vi "[FPGA] DeltaSig Main V6_bis.vi"() -> ()   [LabVIEW 2015]
doc: "This VI provides a template for customizing a waveform acquisition using delta-sigma based NI C Series analog input smodules."
uses:
  <vilib>/LabVIEW Targets/FPGA/cRIO/shared/nicrio_ModuleControls/nicrio_cRIO-9234_ConfigModeRing.ctl
  <vilib>/rvi/Emulation/niFpgaGetClockAttributes.vi
  <vilib>/rvi/Emulation/niFpgaSctlEmulationGetInTimedLoop.vi
  <vilib>/rvi/Emulation/niFpgaEmulationReportErrorSimple.vi
  <vilib>/LabVIEW Targets/FPGA/cRIO/shared/nicrio_DsaDataRateApi/_nicrio_9234GetDataRate131.vi
  <vilib>/rvi/Emulation/niFpgaProcessEmulError.vi
  <vilib>/rvi/eio/common/nirviEmuTemplatePropertySet_errors.vi
  <vilib>/rvi/eio/common/nirviEmuTemplateMethod_errors.vi
  <vilib>/rvi/interface/RandomDataEmulation/niFpgaRandomDataHandleErrors.vi
  <vilib>/rvi/Emulation/niFpgaCriticalErrorInLSC.vi
  <vilib>/eio/EIOPropertyNode/EIOPropertyNode.xnode
  <vilib>/LabVIEW Targets/FPGA/cRIO/shared/nicrio_ModuleControls/nicrio_cRIO-9234_DataRatesRing2.ctl
  <vilib>/eio/EIONode/EIONode.xnode
  <vilib>/rvi/DataTransferAndStorage/Container/XNode/niFpgaContainer.xnode
  <vilib>/rvi/interface/RandomDataEmulation/nirviRandomDataFpgaReadWriteTemplate.vi
  <vilib>/rvi/eio/common/nirviEmuTemplatePropertyGet_errors.vi
  <vilib>/rvi/eio/common/nirviEmuTemplatePropertyGet_noerrors.vi
  <vilib>/rvi/eio/common/nirviEmuTemplatePropertySet_noerrors.vi
panel:
  in  "Array Input Config":T1[](array[typedef])=[0, 0, 0, 0, 0, 0] items=["AC Coupled", "DC Coupled", "IEPE AC Coupled"]
  out "oclk freq":u32
  out "oclk div":u32
  out "oclk mult":u32
  in  "data rate (S/s)":u32
  in  "Chan Scale Array":sgl[](array[numeric])=[0.0, 0.0, 0.0, 0.0, 0.0, 0.0, 0.0, 0.0, 0.0, 0.0, 0.0, 0.0, 0.0, 0.0, 0.0, 0.0, 0.0, 0.0, 0.0, 0.0, 0.0, 0.0, 0.0, 0.0, 0.0, 0.0, 0.0, 0.0, 0.0, 0.0, 0.0, 0.0, 0.0, 0.0, 0.0, 0.0, 0.0, 0.0, 0.0, 0.0]
  out "Chan Count":bool
  out "Acq Loop Ticks":u32
  out "FPGA Error":errorcluster
  out "Module Underflow":bool
  out "Finished":bool
  in  "Number of Channels":i32=24
  in  "Samps per Chan [Finite]":i32=5120
  out "First Read":bool
  in  "Acquisition Type":enum16{"Finite Samples", "Continuous Samples"}(ring)
  out "DMA FIFO Full":bool
  in  "stop":bool
  # "Array size fixed at 40\nelements but may be \nexpanded if needed"
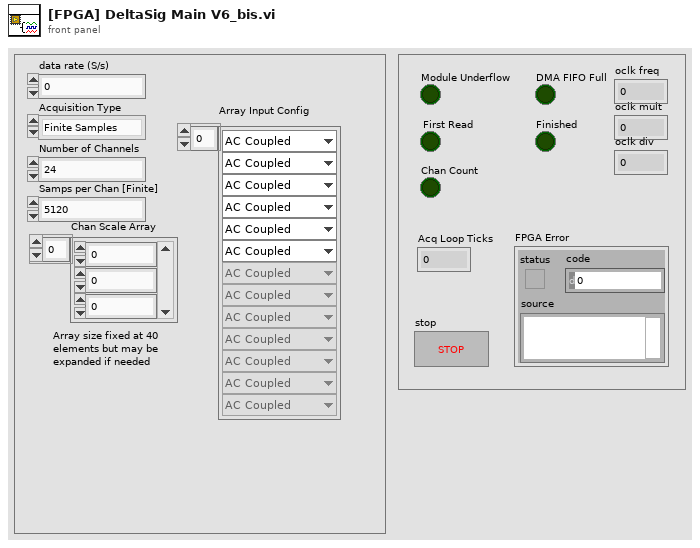
[diagram p1: front panel]
types:
  T1 = typedef "nicrio_cRIO-9234_ConfigModeRing.ctl" = u8
  T2 = typedef "nicrio_cRIO-9234_DataRatesRing2.ctl" = u8
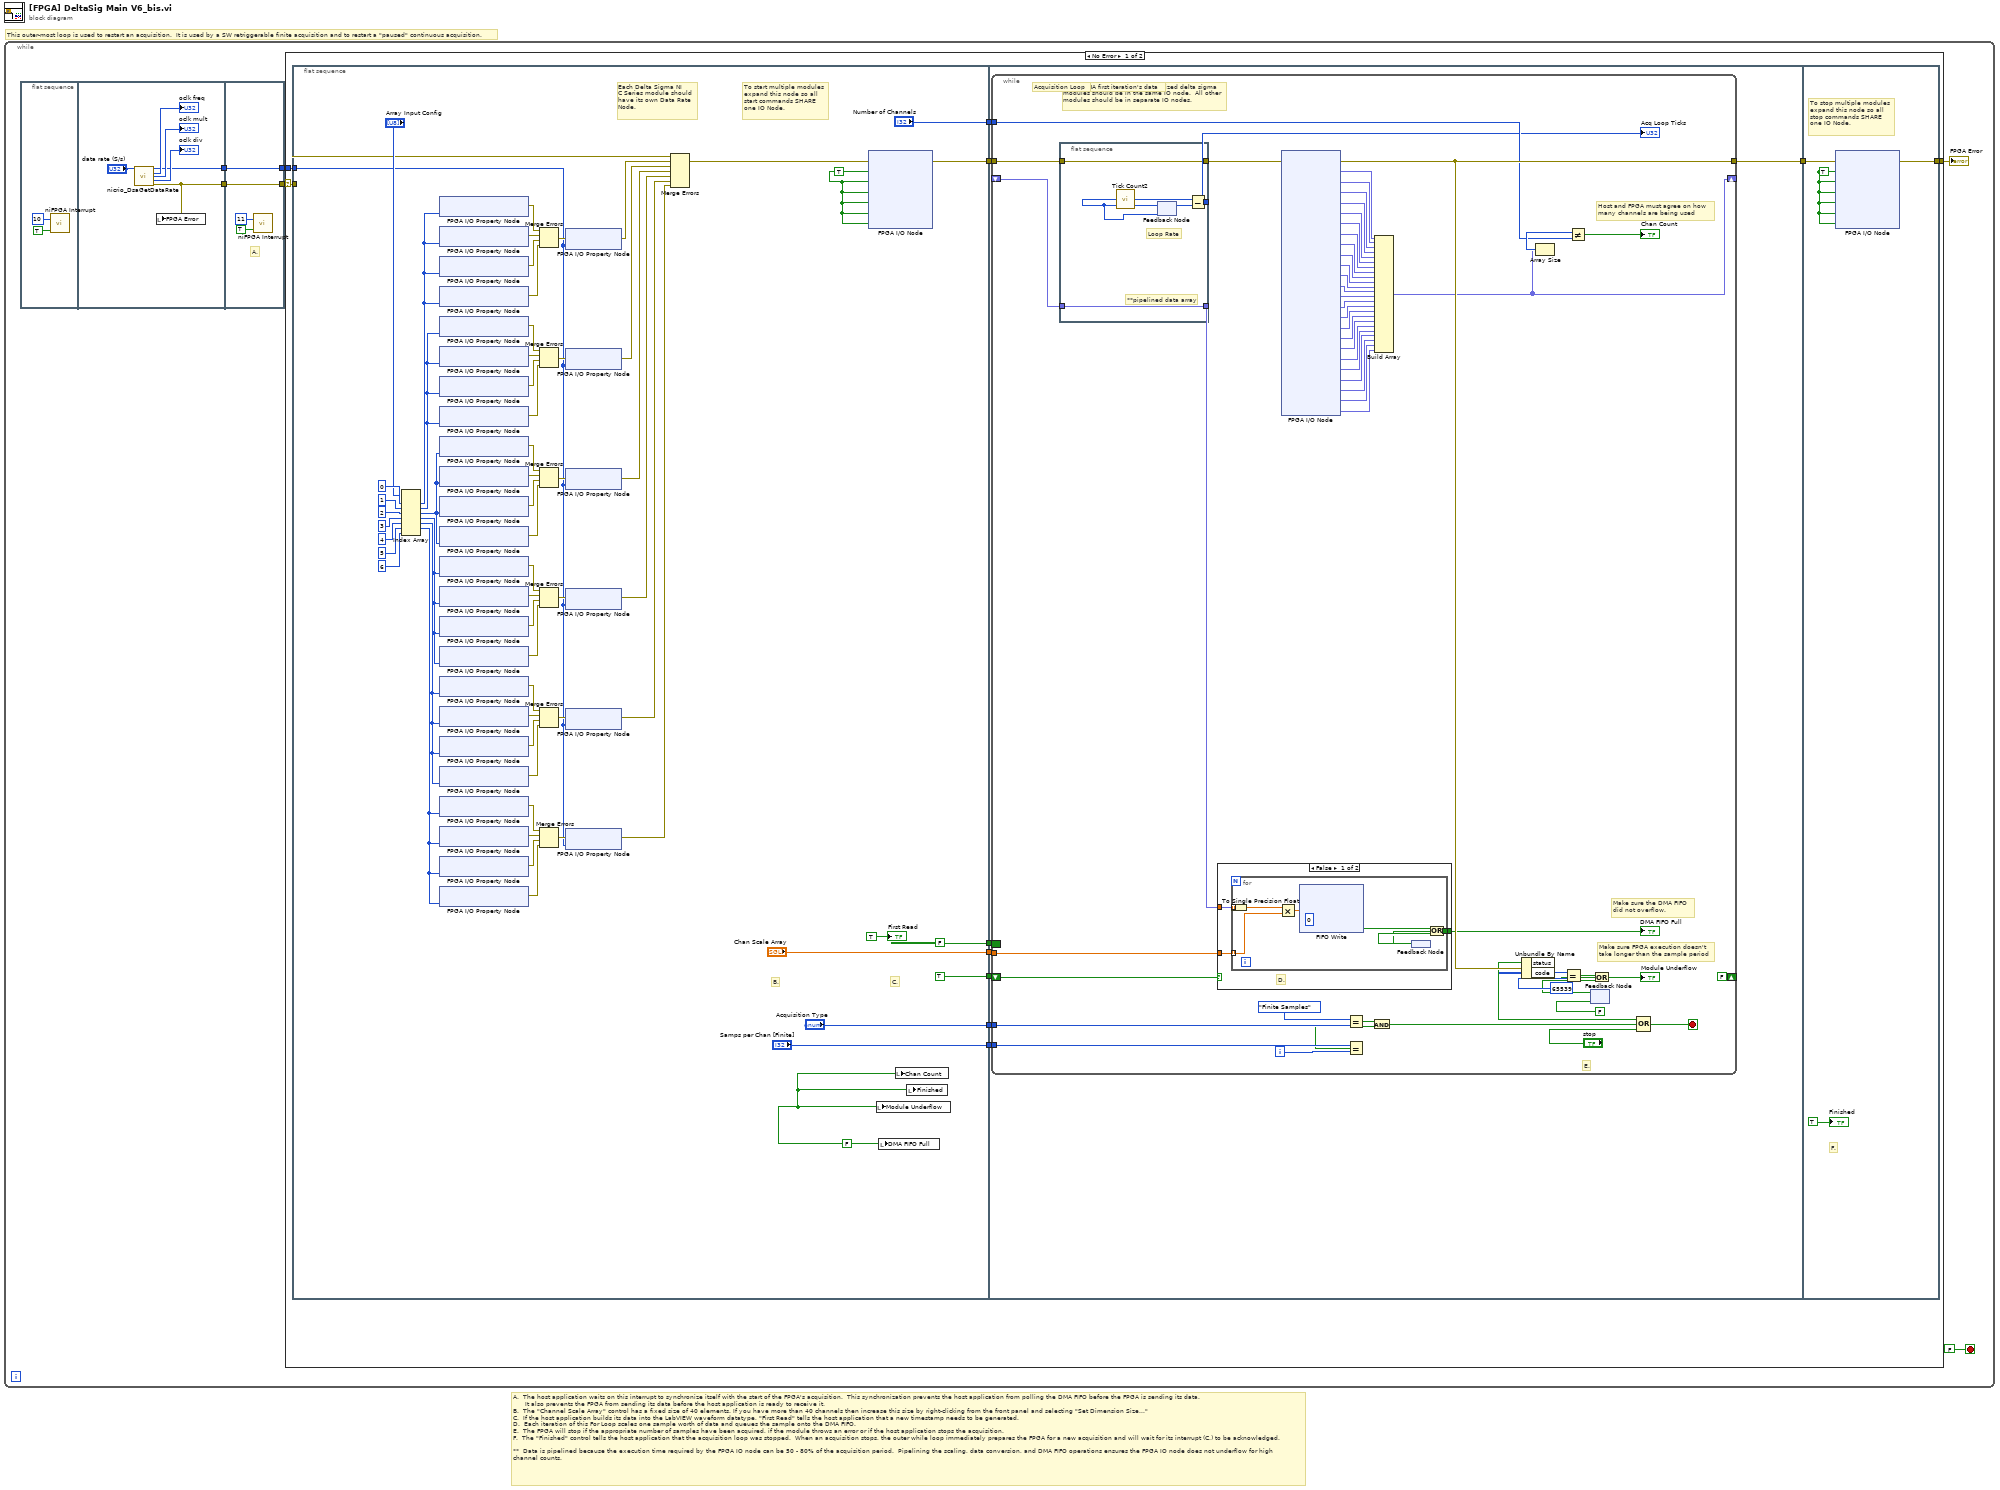
[diagram p0: block diagram]
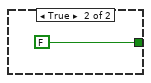
[diagram p2: hidden frame]
diagram:
  # "A.  The host application waits on this interrupt to synchronize itself with the start of the FPGA's acquisition.  This synchronization prevents the host application from polling the DMA FIFO before the FPGA is sending its data.\n      It also prevents the FPGA from sending its data before the host application is ready to receive it.\nB.  The \"Channel Scale Array\" control has a fixed size of 40 elements. If you have more than 40 channels then increase this size by right-clicking from the front panel and selecting \"Set Dimension Size...\"\nC.  If the host application builds its data into the LabVIEW waveform datatype, \"First Read\" tells the host application that a new timestamp needs to be generated.\nD.  Each iteration of this For Loop scales one sample worth of data and queues the sample onto the DMA FIFO.  \nE.  The FPGA will stop if the appropriate number of samples have been acquired, if the module throws an error or if the host application stops the acquisition.  \nF.  The \"Finished\" control tells the host application that the acquisition loop was stopped.  When an acquisition stops, the outer while loop immediately prepares the FPGA for a new acquisition and will wait for its interrupt (C.) to be acknowledged.\n\n**  Data is pipelined because the execution time required by the FPGA IO node can be 50 - 80% of the acquisition period.  Pipelining the scaling, data conversion, and DMA FIFO operations ensures the FPGA IO node does not underflow for high\nchannel counts."
  # "This outer-most loop is used to restart an acquisition.  It is used by a SW retriggerable finite acquisition and to restart a \"paused\" continuous acquisition."
  n1 = while {
    stop <- FALSE stop-if-true
    n2 = flat-sequence {
      tunnel: [w10] -> w2
      tunnel: [w11] -> w1
      tunnel: [w18] -> w3
      tunnel: [w15] -> w4
      tunnel: w2 -> [w15]
      tunnel: w1 -> [w18]
      frame #0 {
        n3 = call <vilib>:"niFPGA Interrupt.vi"("Wait Until Cleared (F)"=TRUE ("Wait Until Cleared"), "IRQ Number (0)"=u8 10 ("IRQ Number")) -> ()  [unwired: 1 in]
      }
      frame #1 {
        n4 = call-poly <vilib>:"nicrio_DsaGetDataRate.vi"("data rate (S/s)"="data rate (S/s)") -> ("data rate"=w11:T2, "oclk freq"=→"oclk freq":u32, "oclk mult"=→"oclk mult":u32, "oclk div"=→"oclk div":u32, "error out"=w10:errorcluster)  [unwired: 10 in]
        n5 = local write "FPGA Error"(w10) -> ()
      }
      frame #2 {
        # "A."
        n6 = call <vilib>:"niFPGA Interrupt.vi"("Wait Until Cleared (F)"=TRUE ("Wait Until Cleared"), "IRQ Number (0)"=u8 11 ("IRQ Number")) -> ()  [unwired: 1 in]
      }
    }
    n7 = case shown="No Error" w4 {
      selector: w4 -> [w19 w176]
      tunnel: [w21 w176] -> w5
      tunnel: w3 -> [w20 _]
      frame No Error {
        n8 = flat-sequence {
          tunnel: [w92] -> w29
          tunnel: ["Chan Scale Array"] -> w28
          tunnel: ["Acquisition Type"] -> w27
          tunnel: ["Samps per Chan [Finite]"] -> w26
          tunnel: ["Number of Channels"] -> w25
          tunnel: [TRUE ("t")] -> w24
          tunnel: [FALSE] -> w23
          tunnel: w20 -> [w38]
          tunnel: w19 -> [w68]
          tunnel: w29 -> [w99]
          tunnel: w28 -> [w98]
          tunnel: w27 -> [w96]
          tunnel: w26 -> [w95]
          tunnel: w25 -> [w100]
          tunnel: w24 -> [w97]
          tunnel: [w94] -> w22
          tunnel: w23 -> [w93]
          tunnel: w22 -> [w174]
          tunnel: [w173] -> w21
          frame #0 {
            w90 = FALSE ("Module Underflow")
            w30 = TRUE ("Mod1/Start")
            # "To start multiple modules\nexpand this node so all\nstart commands SHARE\none IO Node."
            # "C."
            # "B."
            # "Each Delta Sigma NI \nC Series module should \nhave its own Data Rate \nNode."
            n9 = Index Array(array="Array Input Config", index #1=0 ("index"), index #2=1 ("index"), index #3=2 ("index"), index #4=3 ("index"), index #5=4 ("index"), index #6=5 ("index"), index #7=6 ("index")) -> (element #1=w36:T1, element #2=w35:T1, element #3=w34:T1, element #4=w33:T1, element #5=w32:T1, element #6=w31:T1)  [unwired: 1 out]
            n10 = xnode "FPGA I/O Property Node"("Input Configuration"=w36) -> ("error out"=w79:errorcluster)  [unwired: 2 in, 1 out]
            n11 = xnode "FPGA I/O Property Node"("Input Configuration"=w36) -> ("error out"=w78:errorcluster)  [unwired: 2 in, 1 out]
            n12 = xnode "FPGA I/O Property Node"("Input Configuration"=w36) -> ("error out"=w77:errorcluster)  [unwired: 2 in, 1 out]
            n13 = xnode "FPGA I/O Property Node"("Input Configuration"=w36) -> ("error out"=w76:errorcluster)  [unwired: 2 in, 1 out]
            n14 = xnode "FPGA I/O Property Node"("Input Configuration"=w35) -> ("error out"=w73:errorcluster)  [unwired: 2 in, 1 out]
            n15 = xnode "FPGA I/O Property Node"("Input Configuration"=w35) -> ("error out"=w72:errorcluster)  [unwired: 2 in, 1 out]
            n16 = xnode "FPGA I/O Property Node"("Input Configuration"=w35) -> ("error out"=w71:errorcluster)  [unwired: 2 in, 1 out]
            n17 = xnode "FPGA I/O Property Node"("Input Configuration"=w35) -> ("error out"=w70:errorcluster)  [unwired: 2 in, 1 out]
            n18 = xnode "FPGA I/O Property Node"("Input Configuration"=w34) -> ("error out"=w61:errorcluster)  [unwired: 2 in, 1 out]
            n19 = xnode "FPGA I/O Property Node"("Input Configuration"=w34) -> ("error out"=w60:errorcluster)  [unwired: 2 in, 1 out]
            n20 = xnode "FPGA I/O Property Node"("Input Configuration"=w34) -> ("error out"=w59:errorcluster)  [unwired: 2 in, 1 out]
            n21 = xnode "FPGA I/O Property Node"("Input Configuration"=w34) -> ("error out"=w58:errorcluster)  [unwired: 2 in, 1 out]
            n22 = xnode "FPGA I/O Property Node"("Input Configuration"=w33) -> ("error out"=w57:errorcluster)  [unwired: 2 in, 1 out]
            n23 = xnode "FPGA I/O Property Node"("Input Configuration"=w33) -> ("error out"=w56:errorcluster)  [unwired: 2 in, 1 out]
            n24 = xnode "FPGA I/O Property Node"("Input Configuration"=w33) -> ("error out"=w55:errorcluster)  [unwired: 2 in, 1 out]
            n25 = xnode "FPGA I/O Property Node"("Input Configuration"=w33) -> ("error out"=w54:errorcluster)  [unwired: 2 in, 1 out]
            n26 = xnode "FPGA I/O Property Node"("Input Configuration"=w32) -> ("error out"=w53:errorcluster)  [unwired: 2 in, 1 out]
            n27 = xnode "FPGA I/O Property Node"("Input Configuration"=w32) -> ("error out"=w52:errorcluster)  [unwired: 2 in, 1 out]
            n28 = xnode "FPGA I/O Property Node"("Input Configuration"=w32) -> ("error out"=w51:errorcluster)  [unwired: 2 in, 1 out]
            n29 = xnode "FPGA I/O Property Node"("Input Configuration"=w32) -> ("error out"=w50:errorcluster)  [unwired: 2 in, 1 out]
            n30 = xnode "FPGA I/O Property Node"("Input Configuration"=w31) -> ("error out"=w39:errorcluster)  [unwired: 2 in, 1 out]
            n31 = xnode "FPGA I/O Property Node"("Input Configuration"=w31) -> ("error out"=w43:errorcluster)  [unwired: 2 in, 1 out]
            n32 = xnode "FPGA I/O Property Node"("Input Configuration"=w31) -> ("error out"=w42:errorcluster)  [unwired: 2 in, 1 out]
            n33 = xnode "FPGA I/O Property Node"("Input Configuration"=w31) -> ("error out"=w41:errorcluster)  [unwired: 2 in, 1 out]
            n34 = Merge Errors(w79, w78, w77, w76) -> (w75:errorcluster)
            n35 = Merge Errors(w73, w72, w71, w70) -> (w69:errorcluster)
            n36 = Merge Errors(w61, w60, w59, w58) -> (w49:errorcluster)
            n37 = Merge Errors(w57, w56, w55, w54) -> (w48:errorcluster)
            n38 = Merge Errors(w53, w52, w51, w50) -> (w47:errorcluster)
            n39 = Merge Errors(w39, w43, w42, w41) -> (w40:errorcluster)
            n40 = xnode "FPGA I/O Property Node"("error in"=w75, "Data Rate"=w38) -> ("error out"=w66:errorcluster)  [unwired: 1 in, 1 out]
            n41 = xnode "FPGA I/O Property Node"("error in"=w69, "Data Rate"=w38) -> ("error out"=w65:errorcluster)  [unwired: 1 in, 1 out]
            n42 = xnode "FPGA I/O Property Node"("error in"=w49, "Data Rate"=w38) -> ("error out"=w46:errorcluster)  [unwired: 1 in, 1 out]
            n43 = xnode "FPGA I/O Property Node"("error in"=w48, "Data Rate"=w38) -> ("error out"=w45:errorcluster)  [unwired: 1 in, 1 out]
            n44 = xnode "FPGA I/O Property Node"("error in"=w47, "Data Rate"=w38) -> ("error out"=w44:errorcluster)  [unwired: 1 in, 1 out]
            n45 = xnode "FPGA I/O Property Node"("error in"=w40, "Data Rate"=w38) -> ("error out"=w37:errorcluster)  [unwired: 1 in, 1 out]
            n46 = Merge Errors(w68, w66, w65, w46, w45, w44, w37) -> (w67:errorcluster)
            n47 = xnode "FPGA I/O Node"("error in"=w67, "Mod1/Start"=w30, "Mod2/Start"=w30, "Mod3/Start"=w30, "Mod4/Start"=w30, "Mod5/Start"=w30, "Mod6/Start"=w30) -> ("error out"=w92:errorcluster)  [unwired: 6 in, 6 out]
            n48 = local write "Module Underflow"(w90) -> ()
            n49 = local write "DMA FIFO Full"(w90) -> ()
            n50 = local write "Chan Count"(w90) -> ()
            n51 = local write "Finished"(w90) -> ()
            "First Read" <- TRUE ("First Read")
          }
          frame #1 {
            n52 = while {
              tunnel: w99 -> [w144]
              tunnel: [w149] -> w94
              tunnel: w96 -> [w151]
              tunnel: w95 -> [w150]
              shift-right: [w124] -> _
              shift-left: _ -> [w137]
              tunnel: w100 -> [w146]
              tunnel: w98 -> [w138]
              shift-right: [FALSE ("t")] -> _
              shift-left: w97 -> [w136]
              border: w93 -> [_]
              i -> [w134]
              stop <- w121 stop-if-true
              # "Add channels here.  All synchronized delta sigma\nmodules should be in the same IO node.  All other\nmodules should be in separate IO nodes."
              # "Do not DMA first iteration's data"
              # "Acquisition Loop"
              # "E."
              # "Host and FPGA must agree on how \nmany channels are being used"
              # "Make sure the DMA FIFO\ndid not overflow."
              # "Make sure FPGA execution doesn't\ntake longer than the sample period"
              n53 = flat-sequence {
                tunnel: [w171] -> w143
                tunnel: w144 -> [w171]
                tunnel: [w168] -> w142
                tunnel: w137 -> [w167]
                tunnel: [w167] -> w123
                frame #0 {
                  # "**pipelined data array"
                  # "Loop Rate"
                  n54 = call "Tick Count2"() -> ("Tick Count(Ticks)"=w170:u32)
                  n55 = feedback-in #1(w170) -> ()
                  n56 = feedback #1(w170) -> (w169:u32)
                  n57 = Subtract(x=w170, y=w169) -> (x-y=w168:u32)
                }
              }
              n58 = To Single Precision Float(number=w123) -> (single precision float=w122:sgl[])
              n59 = case shown="False" w136 {
                tunnel: [w158 FALSE] -> w148
                tunnel: w138 -> [w157 _]
                tunnel: w122 -> [w156 _]
                frame False {
                  # "D."
                  n60 = for {
                    tunnel: [w163] -> w158
                    tunnel: w156 -> [w161] mode=indexing
                    tunnel: w157 -> [w160] mode=indexing
                    n61 = Multiply(x=w161, y=w160) -> (x*y=w159:sgl)
                    n62 = xnode ("FIFO Write")("Element"=w159, "Timeout"=0) -> ("Timed Out?"=w165:bool)  [unwired: 1 in, 1 out]
                    n63 = feedback #2() -> (w164:bool)
                    n64 = Or(x=w165, y=w164) -> (x .or. y?=w163:bool)
                    n65 = feedback-in #2(w163) -> ()
                  }
                }
                frame True {
                }
              }
              "DMA FIFO Full" <- w148
              n66 = xnode "FPGA I/O Node"("error in"=w143) -> ("error out"=w149:errorcluster, "Mod1/AI0"=w141:fxp<+/-,24,4>, "Mod1/AI1"=w133:fxp<+/-,24,4>, "Mod1/AI2"=w140:fxp<+/-,24,4>, "Mod1/AI3"=w139:fxp<+/-,24,4>, "Mod2/AI0"=w120:fxp<+/-,24,4>, "Mod2/AI1"=w119:fxp<+/-,24,4>, "Mod2/AI2"=w118:fxp<+/-,24,4>, "Mod2/AI3"=w117:fxp<+/-,24,4>, "Mod3/AI0"=w116:fxp<+/-,24,4>, "Mod3/AI1"=w115:fxp<+/-,24,4>, "Mod3/AI2"=w114:fxp<+/-,24,4>, "Mod3/AI3"=w113:fxp<+/-,24,4>, "Mod4/AI0"=w112:fxp<+/-,24,4>, "Mod4/AI1"=w111:fxp<+/-,24,4>, "Mod4/AI2"=w110:fxp<+/-,24,4>, "Mod4/AI3"=w109:fxp<+/-,24,4>, "Mod5/AI0"=w108:fxp<+/-,24,4>, "Mod5/AI1"=w107:fxp<+/-,24,4>, "Mod5/AI2"=w106:fxp<+/-,24,4>, "Mod5/AI3"=w105:fxp<+/-,24,4>, "Mod6/AI0"=w104:fxp<+/-,24,4>, "Mod6/AI1"=w103:fxp<+/-,24,4>, "Mod6/AI2"=w102:fxp<+/-,24,4>, "Mod6/AI3"=w101:fxp<+/-,24,4>)  [unwired: 24 in, 24 out]
              n67 = Equal?(x=enum16{"Finite Samples", "Continuous Samples"}."Finite Samples" ("y"), y=w151) -> (x = y?=w127:bool)
              n68 = Equal?(x=w150, y=w134) -> (x = y?=w126:bool)
              n69 = And(x=w127, y=w126) -> (x .and. y?=w125:bool)
              n70 = Build Array(w141, w133, w140, w139, w120, w119, w118, w117, w116, w115, w114, w113, w112, w111, w110, w109, w108, w107, w106, w105, w104, w103, w102, w101) -> (w124:fxp<+/-,24,4>[])
              n71 = Unbundle By Name(w149) -> ("status"=w132:bool, "code"=w152:i32)
              n72 = Array Size(array=w124) -> (size(s)=w147:i32)
              n73 = Equal?(x=w152, y=65539) -> (x = y?=w129:bool)
              n74 = Not Equal?(x=w147, y=w146) -> (x != y?=→"Chan Count":bool)
              n75 = feedback #3(FALSE) -> (w131:bool)
              n76 = Or(x=w129, y=w131) -> (x .or. y?=w128:bool)
              "Module Underflow" <- w128
              n77 = feedback-in #3(w128) -> ()
              n78 = Compound Arithmetic op=OR(w132, w125, "stop") -> (w121:bool)
              "Acq Loop Ticks" <- w142
            }
          }
          frame #2 {
            w172 = TRUE ("Mod1/Stop")
            # "To stop multiple modules\nexpand this node so all\nstop commands SHARE\none IO Node."
            # "F."
            n79 = xnode "FPGA I/O Node"("error in"=w174, "Mod1/Stop"=w172, "Mod2/Stop"=w172, "Mod3/Stop"=w172, "Mod4/Stop"=w172, "Mod5/Stop"=w172, "Mod6/Stop"=w172) -> ("error out"=w173:errorcluster)  [unwired: 6 in, 6 out]
            "Finished" <- TRUE ("Finished")
          }
        }
      }
      frame Error {
      }
    }
    "FPGA Error" <- w5
  }
